vi "Create Diagnostics Addon.vi"(7 "Configuration (.dat)":path, 8 "error in (no error)":errorcluster, 10 "Name":string, 11 "Custom Devices Ref":refnum<k24>) -> (0 "error out":errorcluster, 3 "Custom Devices Ref":refnum<k24>)   [LabVIEW 2019, in "Diagnostics System Definition API.lvlib"]
uses:
  Diagnostics System Definition API.lvlib
  NationalInstruments.VeriStand.SystemDefinitionAPI
  NationalInstruments.VeriStand.SystemStorage
  Addon/Addon Shared/SubVIs/Constants.vi
  Addon/Addon Shared/Diagnostics Addon Shared.lvlib
  <vilib>/NI/NI VeriStand Custom Device Import and Export Tool/ImportExport.lvlib
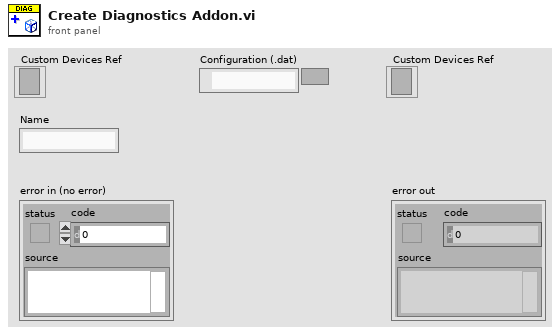
[diagram p1: front panel]
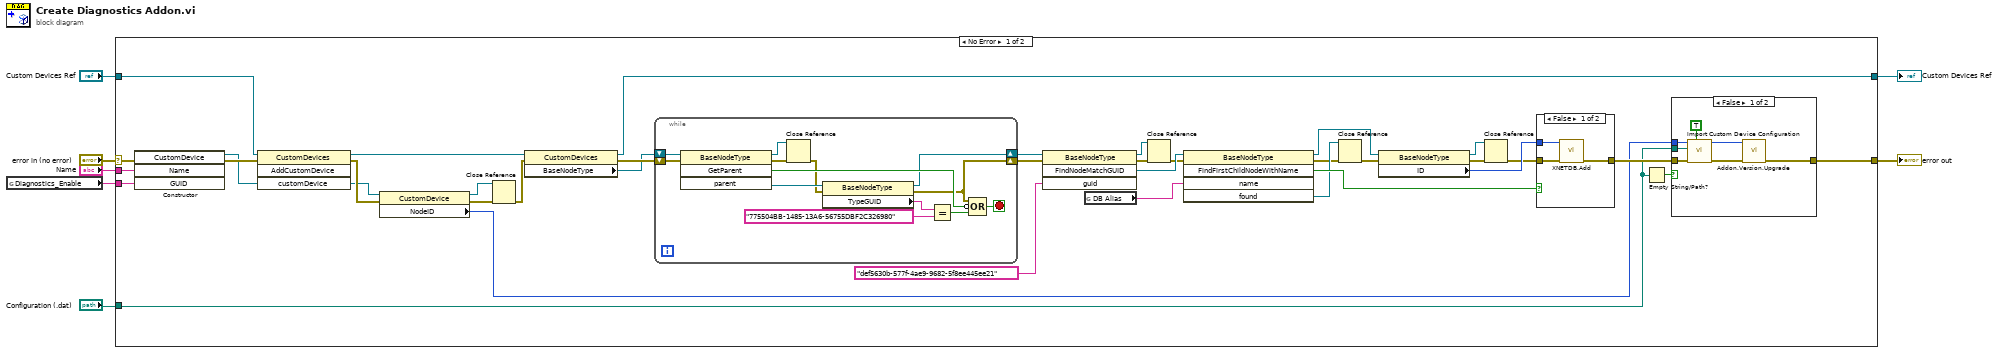
[diagram p0: block diagram]
diagram:
  n1 = global read "Constants.vi" "Diagnostics_Enable"() -> (w7:string)
  n2 = case shown="No Error" "error in (no error)" {
    selector: "error in (no error)" -> [w41 w70]
    tunnel: w7 -> [w43 _]
    tunnel: [w18 w70] -> w6
    tunnel: "Custom Devices Ref" -> [w42 w69]
    tunnel: [w36 w69] -> w4
    tunnel: "Name" -> [w9 _]
    tunnel: "Configuration (.dat)" -> [w8 _]
    frame No Error {
      n3 = constructor class="CustomDevice"(error in=w41, "Name"=w9, "GUID"=w43) -> (reference out=w10:refnum<k24>, error out=w11:errorcluster)  [unwired: 2 in, 3 out]
      n4 = invoke class="CustomDevices" method="AddCustomDevice"(reference=w42, error in=w11, "customDevice"=w10) -> (reference out=w37:refnum<k24>, error out=w16:errorcluster)  [unwired: 1 in, 2 out]
      n5 = property class="CustomDevice"(reference=w10, error in=w16) -> (reference out=w14:refnum<k24>, error out=w15:errorcluster, "NodeID"=w13:u64)
      n6 = Close Reference(reference=w14, error in (no error)=w15) -> (error out=w40:errorcluster)
      n7 = property class="CustomDevices"(reference=w37, error in=w40) -> (reference out=w36:refnum<k24>, error out=w39:errorcluster, "BaseNodeType"=w38:refnum<k24>)
      n8 = while {
        shift-right: [w45] -> w33
        shift-left: w39 -> [w55]
        shift-right: [w44] -> w35
        shift-left: w38 -> [w56]
        stop <- w51 stop-if-true
        n9 = invoke class="BaseNodeType" method="GetParent"(reference=w56, error in=w55) -> (reference out=w46:refnum<k24>, error out=w48:errorcluster, "GetParent"=w52:bool, "parent"=w54:refnum<k24>)  [unwired: 2 in]
        n10 = Close Reference(reference=w46, error in (no error)=w48) -> (error out=w47:errorcluster)
        n11 = property class="BaseNodeType"(reference=w54, error in=w47) -> (reference out=w44:refnum<k24>, error out=w45:errorcluster, "TypeGUID"=w49:string)
        n12 = Equal?(x=w49, y="775504BB-1485-13A6-56755DBF2C326980") -> (x = y?=w53:bool)
        n13 = Compound Arithmetic op=OR(w45, invert w52, w53) -> (w51:bool)
      }
      n14 = invoke class="BaseNodeType" method="FindNodeMatchGUID"(reference=w35, error in=w33, "guid"="def5630b-577f-4ae9-9682-5f8ee445ee21" ("string")) -> (reference out=w32:refnum<k24>, error out=w31:errorcluster, "FindNodeMatchGUID"=w30:refnum<k24>)  [unwired: 1 in, 1 out]
      n15 = global read "Constants.vi" "DB Alias"() -> (w29:string)
      n16 = Close Reference(reference=w32, error in (no error)=w31) -> (error out=w26:errorcluster)
      n17 = invoke class="BaseNodeType" method="FindFirstChildNodeWithName"(reference=w30, error in=w26, "name"=w29) -> (reference out=w27:refnum<k24>, error out=w24:errorcluster, "FindFirstChildNodeWithName"=w28:bool, "found"=w25:refnum<k24>)  [unwired: 2 in, 1 out]
      n18 = Close Reference(reference=w25, error in (no error)=w24) -> (error out=w23:errorcluster)
      n19 = property class="BaseNodeType"(reference=w27, error in=w23) -> (reference out=w21:refnum<k24>, error out=w20:errorcluster, "ID"=w22:u64)
      n20 = Close Reference(reference=w21, error in (no error)=w20) -> (error out=w19:errorcluster)
      n21 = case shown="False" w28 {
        tunnel: [w59 w60] -> w17
        tunnel: w19 -> [w58 w60]
        tunnel: w22 -> [w57 _]
        frame False {
          n22 = call "XNETDB.Add.vi"("error in (no error)"=w58, "Databases Section Ref"=w57) -> ("error out"=w59:errorcluster)  [unwired: 9 in]
        }
        frame True {
        }
      }
      n23 = Empty String/Path?(string/path=w8) -> (empty?=w12:bool)
      n24 = case shown="False" w12 {
        tunnel: [w62 w68] -> w18
        tunnel: w17 -> [w67 w68]
        tunnel: w13 -> [w66 _]
        tunnel: w8 -> [w65 _]
        frame False {
          n25 = call <vilib>:"Import Custom Device Configuration.vi"("Overwrite Existing?"=TRUE, "error in (no error)"=w67, "Path"=w65, "NodeID"=w66) -> ("error out"=w63:errorcluster, "NodeID out"=w61:u64)  [unwired: 5 in, 1 out]
          n26 = call "Addon.Version.Upgrade.vi"("error in (no error)"=w63, "Device Item Ref in in"=w61) -> ("error out"=w62:errorcluster)  [unwired: 8 in, 1 out]
        }
        frame True {
        }
      }
    }
    frame Error {
    }
  }
  "error out" <- w6
  "Custom Devices Ref" <- w4
